vi "Parser_0xEE_(SubVI).vi"(11 "String in":string) -> (0 "substring":string, 1 "Размер описания":i32, 2 "Размер фрагмента":i32, 3 "Смешение в байтах":i32)   [LabVIEW 2017, in "LV_Unicorn.lvlib"]
uses:
  LV_Unicorn.lvlib
panel:
  out "length":i32
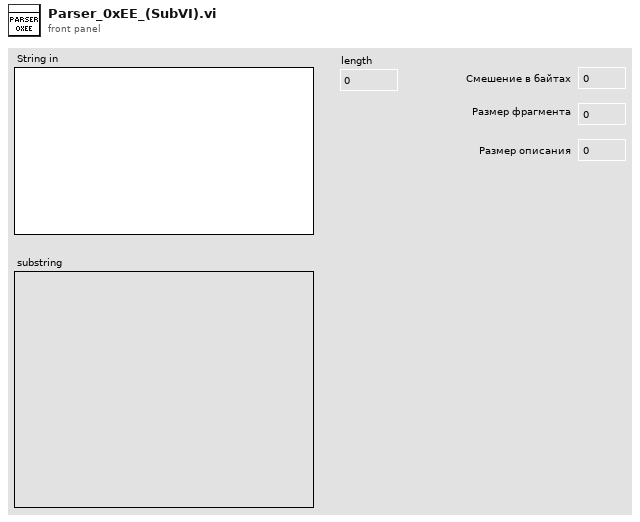
[diagram p1: front panel]
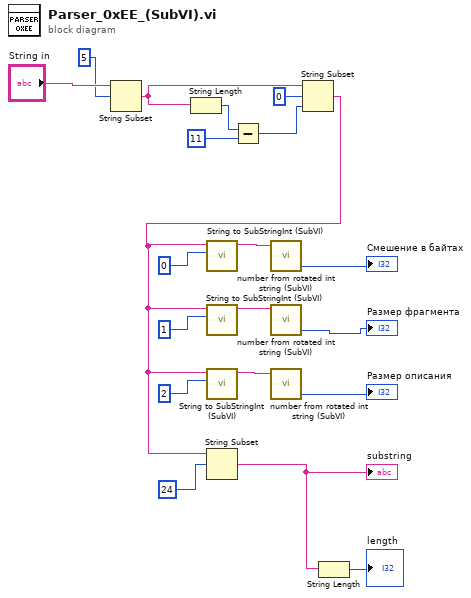
[diagram p0: block diagram]
diagram:
  n1 = String Subset(string="String in", offset (0)=5) -> (substring=w8:string)  [unwired: 1 in]
  n2 = String Length(string=w8) -> (length=w7:i32)
  n3 = Subtract(x=w7, y=11) -> (x-y=w5:i32)
  n4 = String Subset(string=w8, offset (0)=0, length (rest)=w5) -> (substring=w2:string)
  n5 = call "String to SubStringInt (SubVI).vi"("Nx4byte"=u32 0, "String in in"=w2) -> ("String out"=w13:string)  [unwired: 9 in]
  n6 = call "String to SubStringInt (SubVI).vi"("Nx4byte"=u32 1, "String in in"=w2) -> ("String out"=w14:string)  [unwired: 9 in]
  n7 = call "String to SubStringInt (SubVI).vi"("Nx4byte"=u32 2, "String in in"=w2) -> ("String out"=w18:string)  [unwired: 9 in]
  n8 = String Subset(string=w2, offset (0)=24) -> (substring=w1:string)  [unwired: 1 in]
  "substring" <- w1
  n9 = call "number from rotated int string (SubVI).vi"("String"=w13) -> ("int number"=→"Смешение в байтах":i32)  [unwired: 2 in, 2 out]
  n10 = call "number from rotated int string (SubVI).vi"("String"=w14) -> ("int number"=→"Размер фрагмента":i32)  [unwired: 2 in, 2 out]
  n11 = call "number from rotated int string (SubVI).vi"("String"=w18) -> ("int number"=→"Размер описания":i32)  [unwired: 2 in, 2 out]
  n12 = String Length(string=w1) -> (length=→"length":i32)
